vi "Start Cycle.vi"(8 "error in (no error)":errorcluster, 11 "Automation Controller in":refnum<class "Automation Controller.lvclass">) -> (0 "error out":errorcluster, 3 "_State Machine Actor out":refnum<class "_State Machine Actor.lvclass">)   [LabVIEW 2024, in "Automation Controller.lvlib" / "Automation Controller.lvclass"]
uses:
  Automation Controller.lvclass
  Automation Controller.lvclass/Automation Controller.ctl
  C:/Users/uspoaotto/OneDrive - Oregon Tool/Desktop/working copies/stateMachineActor/src/State Machine Actor/State Machine Actor/State Machine Actor.lvclass
  C:/Users/uspoaotto/OneDrive - Oregon Tool/Desktop/working copies/stateMachineActor/src/_State Machine Actor/_State Machine Actor/_State Machine Actor.lvclass
  C:/Program Files (x86)/National Instruments/LabVIEW 2024/vi.lib/ActorFramework/Actor/Actor.lvclass
  C:/Users/uspoaotto/OneDrive - Oregon Tool/Desktop/working copies/stateMachineActor/src/Automation Controller/Automation Controller/Automation Controller.lvclass
  _State Machine Actor/_State Machine Actor/_State Machine Actor.lvclass
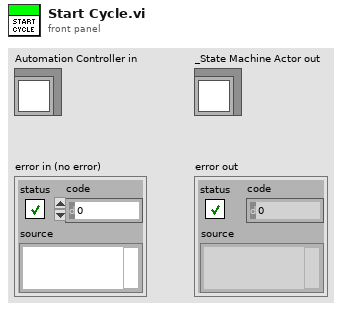
[diagram p1: front panel]
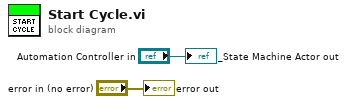
[diagram p0: block diagram]
diagram:
  "error out" <- "error in (no error)"
  "_State Machine Actor out" <- "Automation Controller in"
